vi "Construct Notifier Transport.vi"() -> (0 "error out":errorcluster, 3 "NotifierTransport":refnum<class "NotifierTransport.lvclass">)   [LabVIEW 2018, in "MVA Framework.lvlib" / "NotifierTransport.lvclass"]
doc: "构建通知器传输"
uses:
  NotifierTransport.lvclass
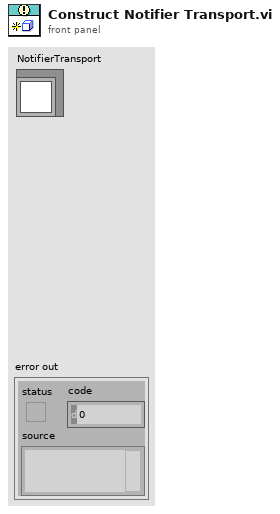
[diagram p1: front panel]
types:
  T1 = cluster{"Data":variant, "Publication Time":timestamp}
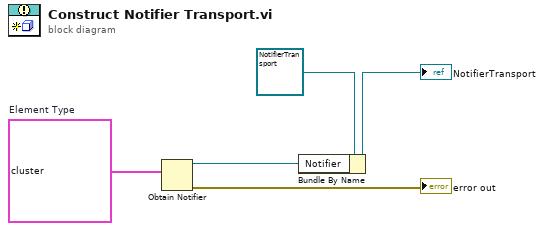
[diagram p0: block diagram]
diagram:
  w3 = T1 {"Data"=variant, "Publication Time"=timestamp(0 s since 1904-01-01)}  # Element Type
  n1 = Obtain Notifier(notification data type=w3) -> (notifier out=w1:refnum<notifier>, error out=→"error out":errorcluster)  [unwired: 3 in, 1 out]
  n2 = Bundle By Name(cluster=refnum<class "NotifierTransport.lvclass"> refnum ("QueueTransport.lvclass"), "Notifier"=w1) -> (→"NotifierTransport":refnum<class "NotifierTransport.lvclass">)
